vi "SubVI_COP_R.vi"(3 "Filtered x in":dbl, 4 "Filtered x in":dbl, 5 "Filtered x out 3":dbl, 6 "Filtered x out 4":dbl) -> (0 "Sum Left":dbl, 1 "Y Left":dbl, 2 "X Left":dbl)   [LabVIEW 2019]
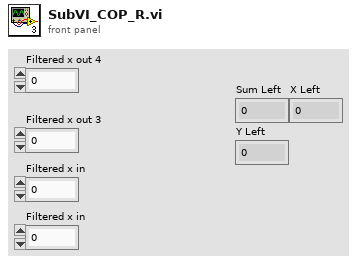
[diagram p1: front panel]
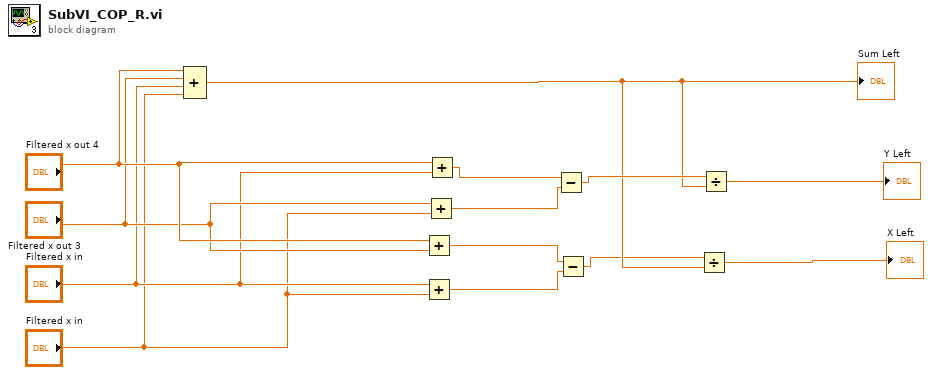
[diagram p0: block diagram]
diagram:
  n1 = Compound Arithmetic op=ADD("Filtered x out 4", "Filtered x out 3", "Filtered x in", "Filtered x in") -> (w4:dbl)
  "Sum Left" <- w4
  n2 = Add(x="Filtered x out 4", y="Filtered x out 3") -> (x+y=w7:dbl)
  n3 = Add(x="Filtered x in", y="Filtered x in") -> (x+y=w6:dbl)
  n4 = Add(x="Filtered x out 3", y="Filtered x in") -> (x+y=w8:dbl)
  n5 = Add(x="Filtered x out 4", y="Filtered x in") -> (x+y=w9:dbl)
  n6 = Subtract(x=w9, y=w8) -> (x-y=w5:dbl)
  n7 = Subtract(x=w7, y=w6) -> (x-y=w3:dbl)
  n8 = Divide(x=w3, y=w4) -> (x/y=→"X Left":dbl)
  n9 = Divide(x=w5, y=w4) -> (x/y=→"Y Left":dbl)
